vi "Attenuator Check Calibration From INI File.vi"(7 "Paramters to Measure":T6[](array[typedef]) {"Channel" min=1 max=99 step=1; "Parameter"."Stimulus Port" min=1 step=1; "Parameter"."Response Port" min=1 step=1}, 8 "error in (no error)":errorcluster, 11 "Requested Stimulus":T1={"ATT Stimulus"={"Normalize"=TRUE, "Value (dB)"=0.0}, "VNA Stimulus"={"Use Instrument Settings"=FALSE, "Blank Frequencies"=FALSE, "Sweep Type"=enum."Linear", "Sweep"={"Fstart"=500.0, "Fstop"=1500.0, "Units"=enum."MHz", "Points"=201}, "Power (dBm)"=999.0, "IFBW (Hz)"=-1.0, "Sweep Time (s)"=-1.0, "Calibration"={"State"=FALSE, "String"=""}}} {"VNA Stimulus"."Sweep Time (s)" format="%.3g"}) -> (0 "error out":errorcluster, 1 "Check Instrument":bool, 3 "Stimulus Out":T1={"ATT Stimulus"={"Normalize"=TRUE, "Value (dB)"=0.0}, "VNA Stimulus"={"Use Instrument Settings"=FALSE, "Blank Frequencies"=FALSE, "Sweep Type"=enum."Linear", "Sweep"={"Fstart"=500.0, "Fstop"=1500.0, "Units"=enum."MHz", "Points"=201}, "Power (dBm)"=999.0, "IFBW (Hz)"=-1.0, "Sweep Time (s)"=-1.0, "Calibration"={"State"=FALSE, "String"=""}}} {"VNA Stimulus"."Sweep Time (s)" format="%.3g"}, 5 "Paramters to Measure Out":T6[](array[typedef]) {"Channel" min=1 max=99 step=1; "Parameter"."Stimulus Port" min=1 step=1; "Parameter"."Response Port" min=1 step=1})   [LabVIEW 2011]
uses:
  TypeDefs/Attenuator Parameter to Measure.ctl
  S Parameter/TypeDefs/SP Parameter.ctl
  TypeDefs/Attenuator VNA Calibration State.ctl
  S Parameter/TypeDefs/SP Measurement Format.ctl
  TypeDefs/Attenuator Stimulus Parameters.ctl
  TypeDefs/Attenuator ATT Stimulus.ctl
  TypeDefs/Attenuator VNA Stimulus.ctl
  S Parameter/TypeDefs/SP Frequency Units.ctl
  Summitek EXT/OpenG EXT/file/file.llb/File Exists - Scalar__ogtk.vi
  <vilib>/Utility/config.llb/Read Key (String).vi
  <vilib>/Utility/config.llb/NI_LVConfig.lvlib
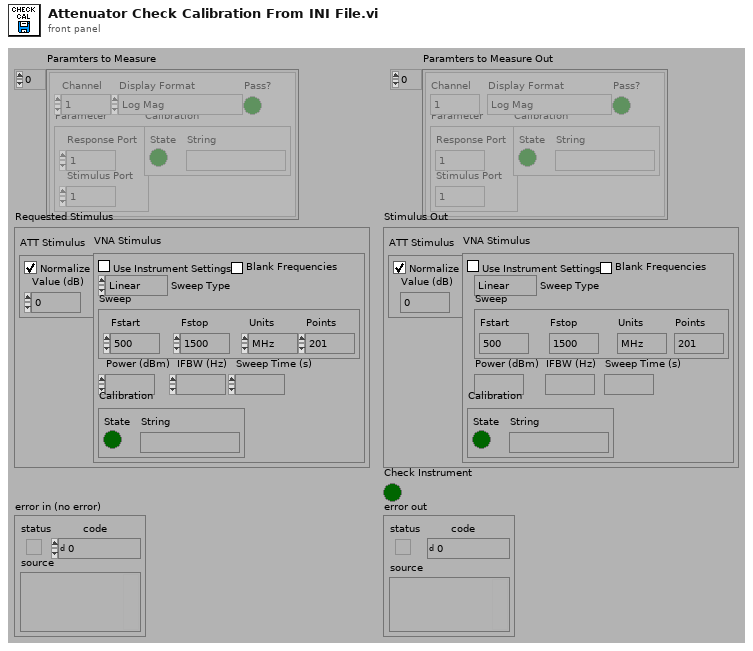
[diagram p1: front panel]
types:
  T1 = typedef "Attenuator Stimulus Parameters.ctl" = cluster{"ATT Stimulus":T2, "VNA Stimulus":T3}
  T2 = typedef "Attenuator ATT Stimulus.ctl" = cluster{"Normalize":bool, "Value (dB)":dbl}
  T3 = typedef "Attenuator VNA Stimulus.ctl" = cluster{"Use Instrument Settings":bool, "Blank Frequencies":bool, "Sweep Type":enum32{"Linear", "Logarithmic", "List", "Power", "CW"}, "Sweep":cluster{"Fstart":dbl, "Fstop":dbl, "Units":T4, "Points":i32}, "Power (dBm)":dbl, "IFBW (Hz)":dbl, "Sweep Time (s)":dbl, "Calibration":T5}
  T4 = typedef "SP Frequency Units.ctl" = enum16{"Hz", "kHz", "MHz", "GHz", "Points"}
  T5 = typedef "Attenuator VNA Calibration State.ctl" = cluster{"State":bool, "String":string}
  T6 = typedef "Attenuator Parameter to Measure.ctl" = cluster{"Channel":i8, "Parameter":T7, "Calibration":T5, "Display Format":T8, "Pass?":bool}
  T7 = typedef "SP Parameter.ctl" = cluster{"Stimulus Port":i8, "Response Port":i8}
  T8 = typedef "SP Measurement Format.ctl" = enum32{"Log Mag", "Phase", "Delay", "Smith (R+jX)", "Polar (Re/Im)", "Linear Mag", "SWR", "Real", "Imaginary", "Smith (Lin/Phase)", "Smith (Log/Phase)", "Smith (Real/Imag)", "Smith (G+jB)", "Polar (Lin/Phase)", "Polar (Log/Phase)", "Expanded Phase", "Positive Phase", "Inverted Smith", "Unwrapped Phase", "Power Out", "Power In", "Linear Mag/Phase", "Log Mag/Phase", "Real/Imaginary"}
  T9 = typedef "NI_LVConfig.lvlib/Config Data RefNum.ctl" = refnum<k1>
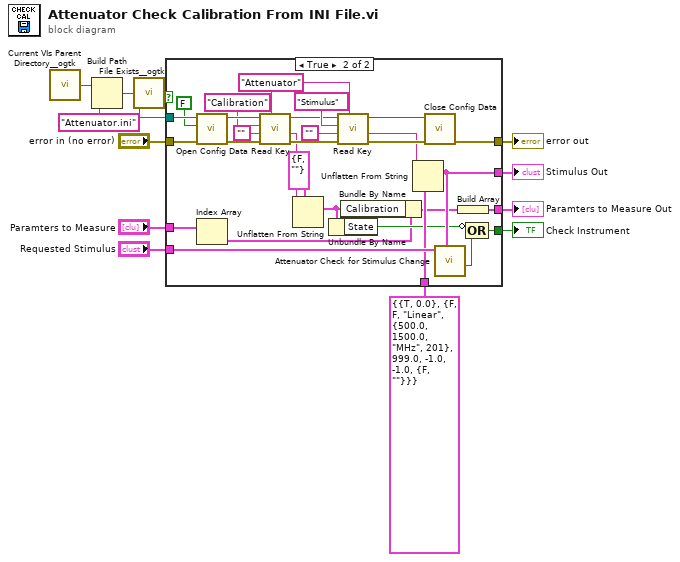
[diagram p0: block diagram]
diagram:
  n1 = call "Current VIs Parent Directory__ogtk.vi"() -> ("Parent Directory (+ Relative)"=w5:path)  [unwired: 5 in]
  n2 = Build Path(base path=w5, name or relative path="Attenuator.ini") -> (appended path=w2:path)
  n3 = call-poly "File Exists__ogtk.vi"("file path"=w2) -> ("exists"=w4:bool)  [unwired: 6 in, 1 out]
  n4 = case shown="True" w4 {
    selector: w4 -> [w13 _]
    tunnel: "error in (no error)" -> [_ w42]
    tunnel: [_ w38] -> w10
    tunnel: w2 -> [_ w41]
    tunnel: [w13 w16] -> w11
    tunnel: "Requested Stimulus" -> [_ w40]
    tunnel: "Paramters to Measure" -> [_ w21]
    tunnel: T1 {"ATT Stimulus"={"Normalize"=TRUE, "Value (dB)"=0.0}, "VNA Stimulus"={"Use Instrument Settings"=FALSE, "Blank Frequencies"=FALSE, "Sweep Type"=enum."Linear", "Sweep"={"Fstart"=500.0, "Fstop"=1500.0, "Units"=enum."MHz", "Points"=201}, "Power (dBm)"=999.0, "IFBW (Hz)"=-1.0, "Sweep Time (s)"=-1.0, "Calibration"={"State"=FALSE, "String"=""}}} ("Attenuator Stimulus") -> [_ w33]
    tunnel: [_ w14] -> w1
    tunnel: [_ w27] -> w6
    frame False {
    }
    frame True {
      w26 = "Attenuator" ("name or relative path")
      n5 = call <vilib>:"Open Config Data.vi"("error in (no error)"=w42, "create file if necessary (T)"=FALSE ("create file if necessary? (T)"), "configuration file path"=w41) -> ("error out"=w32:errorcluster, "refnum"=w31:T9)  [unwired: 6 in, 1 out]
      n6 = Index Array(array=w21) -> (element=w18:T6)  [unwired: 1 in]
      n7 = call-poly <vilib>:"Read Key.vi"("section"=w26, "error in (no error)"=w32, "default value"="", "key"="Calibration" ("format string"), "refnum"=w31) -> ("error out"=w30:errorcluster, "value"=w24:string, "refnum out"=w29:T9)  [unwired: 1 in, 3 out]
      n8 = Unflatten From String(type=T5 {"State"=FALSE, "String"=""} ("Calibration State"), binary string=w24) -> (value=w22:T5)  [unwired: 1 in, 4 out]
      n9 = Unbundle By Name(w22) -> ("State"=w19:bool)
      n10 = call-poly <vilib>:"Read Key.vi"("section"=w26, "error in (no error)"=w30, "default value"="", "key"="Stimulus", "refnum"=w29) -> ("error out"=w39:errorcluster, "value"=w34:string, "refnum out"=w37:T9)  [unwired: 1 in, 3 out]
      n11 = Bundle By Name(cluster=w18, "Calibration"=w22) -> (w15:T6)
      n12 = Unflatten From String(type=w33, binary string=w34) -> (value=w27:T1)  [unwired: 1 in, 4 out]
      n13 = call <vilib>:"Close Config Data.vi"("error in (no error)"=w39, "refnum"=w37) -> ("error out"=w38:errorcluster)  [unwired: 1 in, 8 out]
      n14 = call "Attenuator Check for Stimulus Change.vi"("Current Stimulus Channel"=w27, "New Stimulus"=w40) -> ("Stimulus Changed?"=w17:bool)  [unwired: 7 in, 2 out]
      n15 = Build Array(w15) -> (w14:T6[])
      n16 = Compound Arithmetic op=OR(invert w19, w17) -> (w16:bool)
    }
  }
  "error out" <- w10
  "Check Instrument" <- w11
  "Paramters to Measure Out" <- w1
  "Stimulus Out" <- w6
